vi "TRACK 1 of N USING C.vi"(0 "starting x 1":i16=90, 1 "starting y 1":i16=90, 2 "Calibration cluster 1":T1={"forget radius"=10, "z step"=0.10000000149011612, "cosine bandpass"=[0.0+0.0i, 0.0+0.0i, 0.0+0.0i, 0.0+0.0i, 0.0+0.0i, 0.0+0.0i, 0.013477564910012285+0.0i, 0.05318368061643486+0.0i, 0.11697778011223647+0.0i, 0.20142070693009556+0.0i, 0.30196009946809654+0.0i, 0.41317591628899897+0.0i, 0.5290723971462832+0.0i, 0.6434016229995044+0.0i, 0.7500000270277161+0.0i, 0.8431207911892551+0.0i, 0.9177438980844319+0.0i, 0.9698463139509803+0.0i, 0.9966191828966751+0.0i, 0.9966191828966752+0.0i, 0.9698462819287371+0.0i, 0.917743898084432+0.0i, 0.8431208592908894+0.0i, 0.7499999459445649+0.0i, 0.6434016229995043+0.0i, 0.5290724906146382+0.0i, 0.41317587018682134+0.0i, 0.301960142452895+0.0i, 0.20142063182990733+0.0i, 0.1169777650667072+0.0i, 0.05318370162624281+0.0i, 0.013477548716154919+0.0i, 0.0+0.0i, 0.0+0.0i, 0.0+0.0i, 0.0+0.0i, 0.0+0.0i, 0.0+0.0i, 0.0+0.0i, 0.0+0.0i, 0.0+0.0i, 0.0+0.0i, 0.0+0.0i, 0.0+0.0i, 0.0+0.0i, 0.0+0.0i, 0.0+0.0i, 0.0+0.0i, 0.0+0.0i, 0.0+0.0i, 0.0+0.0i, 0.0+0.0i, 0.0+0.0i, 0.0+0.0i, 0.0+0.0i, 0.0+0.0i, 0.0+0.0i, 0.0+0.0i, 0.0+0.0i, 0.0+0.0i, 0.0+0.0i, 0.0+0.0i, 0.0+0.0i, 0.0+0.0i, 0.0+0.0i, 0.0+0.0i, 0.0+0.0i, 0.0+0.0i, 0.0+0.0i, 0.0+0.0i, 0.0+0.0i, 0.0+0.0i, 0.0+0.0i, 0.0+0.0i, 0.0+0.0i, 0.0+0.0i, 0.0+0.0i, 0.0+0.0i, 0.0+0.0i, 0.0+0.0i, 0.0+0.0i, 0.0+0.0i, 0.0+0.0i, 0.0+0.0i, 0.0+0.0i, 0.0+0.0i, 0.0+0.0i, 0.0+0.0i, 0.0+0.0i, 0.0+0.0i, 0.0+0.0i, 0.0+0.0i, 0.0+0.0i, 0.0+0.0i, 0.0+0.0i, 0.0+0.0i, 0.0+0.0i, 0.0+0.0i, 0.0+0.0i, 0.0+0.0i, 0.0+0.0i, 0.0+0.0i, 0.0+0.0i, 0.0+0.0i, 0.0+0.0i, 0.0+0.0i, 0.0+0.0i, 0.0+0.0i, 0.0+0.0i, 0.0+0.0i, 0.0+0.0i, 0.0+0.0i, 0.0+0.0i, 0.0+0.0i, 0.0+0.0i, 0.0+0.0i, 0.0+0.0i, 0.0+0.0i, 0.0+0.0i, 0.0+0.0i, 0.0+0.0i, 0.0+0.0i, 0.0+0.0i, 0.0+0.0i, 0.0+0.0i, 0.0+0.0i, 0.0+0.0i, 0.0+0.0i], "2D array of prepped\ncal image amplitudes\nr shifted!"=array10x54[540 elements], "2D array of complex\ncal image intensities\n(aka cal corkscrews)\nr shifted!"=array10x54[540 elements], "Real portion of\nhilbert/bandpass filtered\nr-shifted claibration image"=array10x54[540 elements]} {"Real portion of\nhilbert/bandpass filtered\nr-shifted claibration image" format="%.2f"; "2D array of complex\ncal image intensities\n(aka cal corkscrews)\nr shifted!" format="%.2f"; "2D array of prepped\ncal image amplitudes\nr shifted!" format="%.2f"; "cosine bandpass" format="%.2f"}, 3 "Bead 1 is good? in":bool=TRUE, 10 "Image Pixels (Float)":sgl[][](array[numeric])=array180x180[32400 elements] format="%.2f", 12 "cross size":i32=128) -> (16 "Bead 1 is good? out":bool=TRUE, 18 "Index of closest\ncal image slice, bead 1":i32, 20 "X pos 1":dbl format="%.2f", 21 "Y pos 1":dbl format="%.2f", 22 "Z pos 1":dbl, 23 "bead 1 z position\nas a cal image index":dbl format="%.2f")   [LabVIEW 2014]
uses:
  x64/Release/CPU Tracking.dll
panel:
  out "error out":errorcluster
  in  "Cross Thickness":i32=10
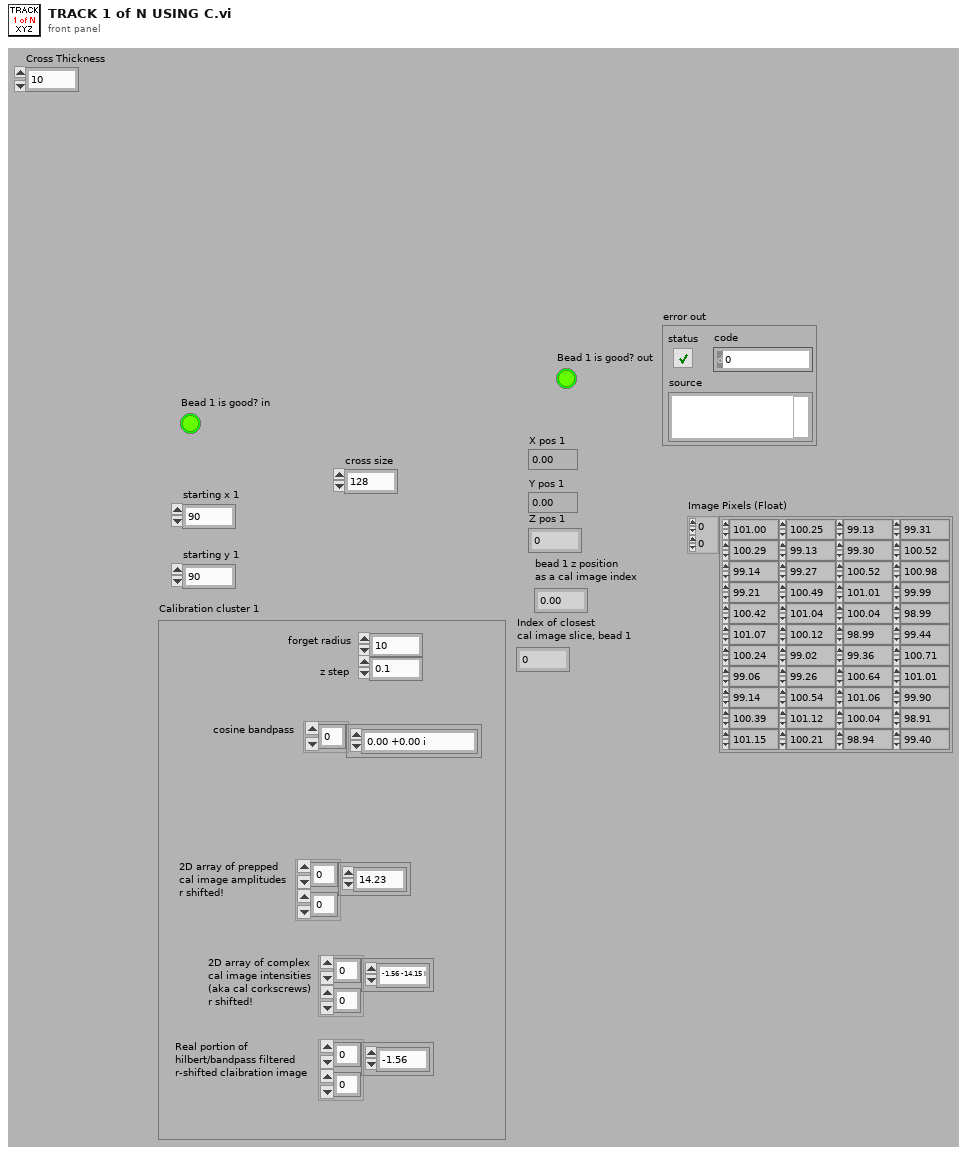
[diagram p1: front panel]
types:
  T1 = cluster{"forget radius":i32, "z step":dbl, "cosine bandpass":cdb[], "2D array of prepped\ncal image amplitudes\nr shifted!":dbl[][], "2D array of complex\ncal image intensities\n(aka cal corkscrews)\nr shifted!":cdb[][], "Real portion of\nhilbert/bandpass filtered\nr-shifted claibration image":dbl[][]}
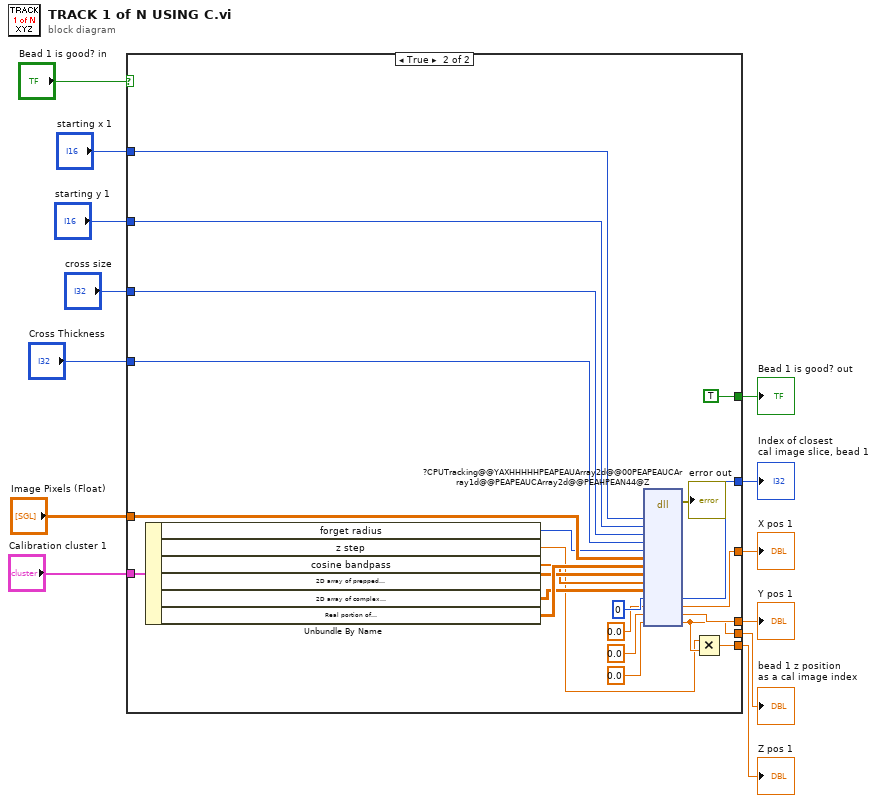
[diagram p0: block diagram]
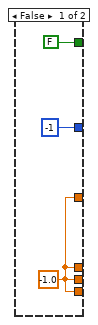
[diagram p2: hidden frame]
diagram:
  n1 = case shown="True" "Bead 1 is good? in" {
    tunnel: [w15 w26] -> w13
    tunnel: "Calibration cluster 1" -> [_ w39]
    tunnel: [-1 ("Index of closest\ncal image slice") w30] -> w11
    tunnel: "starting x 1" -> [_ w22]
    tunnel: "starting y 1" -> [_ w21]
    tunnel: [w15 w32] -> w8
    tunnel: [w15 w31] -> w7
    tunnel: [w15 w28] -> w6
    tunnel: [FALSE TRUE] -> w5
    tunnel: "cross size" -> [_ w20]
    tunnel: "Image Pixels (Float)" -> [_ w37]
    tunnel: "Cross Thickness" -> [_ w19]
    frame False {
      w15 = -1.0 ("new profile\ncenter")
    }
    frame True {
      n2 = Unbundle By Name(w39) -> ("forget radius"=w18:i32, "z step"=w27:dbl, "cosine bandpass"=w34:cdb[], "2D array of prepped\ncal image amplitudes\nr shifted!"=w35:dbl[][], "2D array of complex\ncal image intensities\n(aka cal corkscrews)\nr shifted!"=w33:cdb[][], "Real portion of\nhilbert/bandpass filtered\nr-shifted claibration image"=w36:dbl[][])
      n3 = dll-call lib="D:/LV-SVN/Projects/Bob/GPU Tracking Demo/CPU Tracking & Calibration/x64/Release/CPU Tracking.dll" fn="?CPUTracking@@YAXHHHHHPEAPEAUArray2d@@00PEAPEAUCArray1d@@PEAPEAUCArray2d@@PEAHPEAN44@Z"("Start X"=w22, "Start Y"=w21, "Cross"=w20, "Cross Thickness"=w19, "Forget Radius"=w18, "Image"=w37, "Real Portin of Calibration"=w36, "Cal Image Amplitudes"=w35, "Cos Bandpass"=w34, "Corkscrews"=w33, "Best Fit Index"=0, "New X"=0.0 ("New Y"), "New Y"=0.0, "Z Position"=0.0 ("New Y")) -> (error out=→"error out":errorcluster, "Best Fit Index"=w30:i32, "New X"=w32:dbl, "New Y"=w31:dbl, "Z Position"=w28:dbl)  [unwired: 14 in, 1 out]
      n4 = Multiply(x=w27, y=w28) -> (x*y=w26:dbl)
    }
  }
  "Index of closest\ncal image slice, bead 1" <- w11
  "Z pos 1" <- w13
  "X pos 1" <- w8
  "Y pos 1" <- w7
  "bead 1 z position\nas a cal image index" <- w6
  "Bead 1 is good? out" <- w5
